vi "Email to Handler.vi"(7 "Email Mode":T1, 8 "Email Handler IP":string, 9 "Message:":string, 10 "Subject:":string, 11 "To:":string) -> ()   [LabVIEW 2013]
uses:
  Controls/Email Mode.ctl
panel:
  out "error out":errorcluster
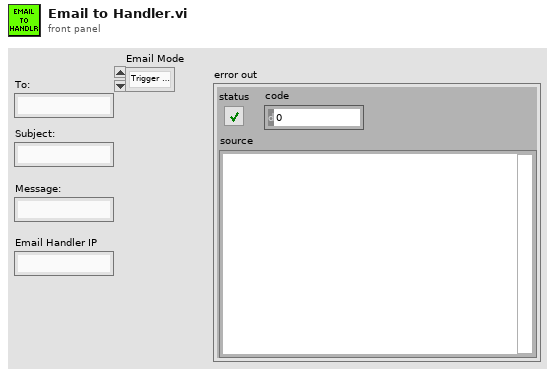
[diagram p1: front panel]
types:
  T1 = typedef "Email Mode.ctl" = enum16{"Trigger Email", "Send Email"}
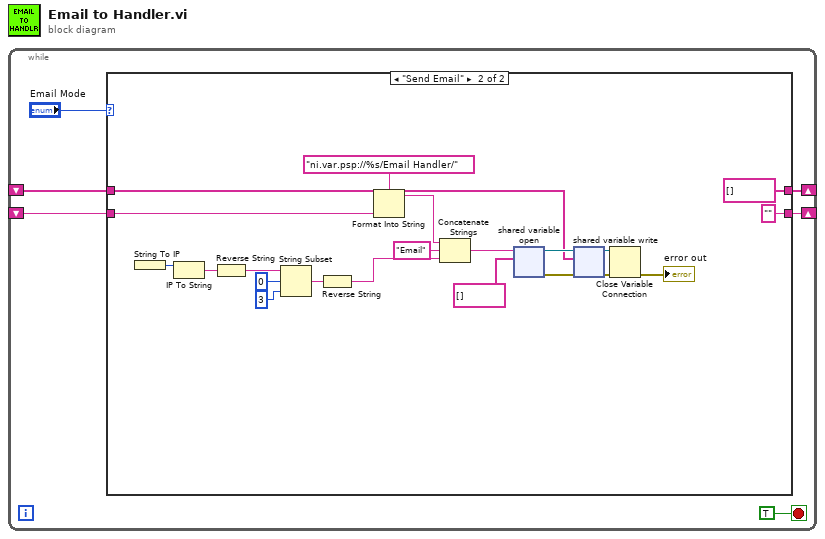
[diagram p0: block diagram]
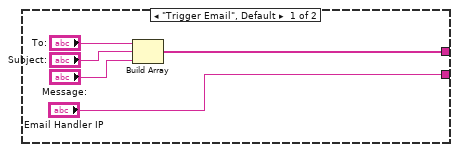
[diagram p2: hidden frame]
diagram:
  n1 = while {
    shift-right: [w4] -> _
    shift-left: _ -> [w1]
    shift-right: [w3] -> _
    shift-left: _ -> [w2]
    stop <- TRUE stop-if-true
    n2 = case shown="\"Send Email\"" "Email Mode" {
      tunnel: [w8 string[] []] -> w4
      tunnel: ["Email Handler IP" "" ("Email Handler IP")] -> w3
      tunnel: w2 -> [_ w15]
      tunnel: w1 -> [_ w14]
      frame "Trigger Email", Default {
        n3 = Build Array("To:", "Subject:", "Message:") -> (w8:string[])
      }
      frame "Send Email" {
        n4 = String To IP() -> (0:w30:u32)  [unwired: 1 in]
        n5 = IP To String(2:w30) -> (0:w29:string)  [unwired: 1 in]
        n6 = Reverse String(1:w29) -> (0:w27:string)
        n7 = String Subset(string=w27, offset (0)=0, length (rest)=3 ("length (rest)")) -> (substring=w26:string)
        n8 = Reverse String(1:w26) -> (0:w25:string)
        n9 = Format Into String(format string="ni.var.psp://%s/Email Handler/", w15) -> (resulting string=w17:string)  [unwired: 2 in, 1 out]
        n10 = Concatenate Strings(w17, "Email" ("string"), w25) -> (w16:string)
        n11 = shared-variable-open(w16, string[] []) -> (w23:refnum<k21>, w21:errorcluster)  [unwired: 2 in]
        n12 = shared-variable-write(w23, w21, w14) -> (w24:refnum<k21>, w22:errorcluster)
        n13 = Close Variable Connection(8:w22, 11:w24) -> (0:→"error out":errorcluster)
      }
    }
  }
